vi "dB_autoselector.vi"(8 "error_in":errorcluster, 11 "Amplitude":dbl) -> (0 "error_out":errorcluster, 3 "Attenuator(dB)":T1)   [LabVIEW 2017]
uses:
  controls/attenuator_dB.ctl
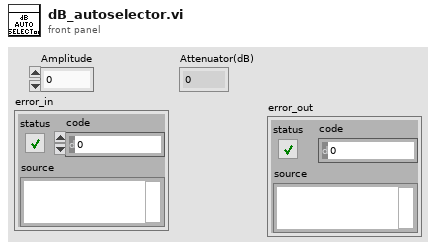
[diagram p1: front panel]
types:
  T1 = typedef "attenuator_dB.ctl" = enum16{"0", "20", "40", "60"}
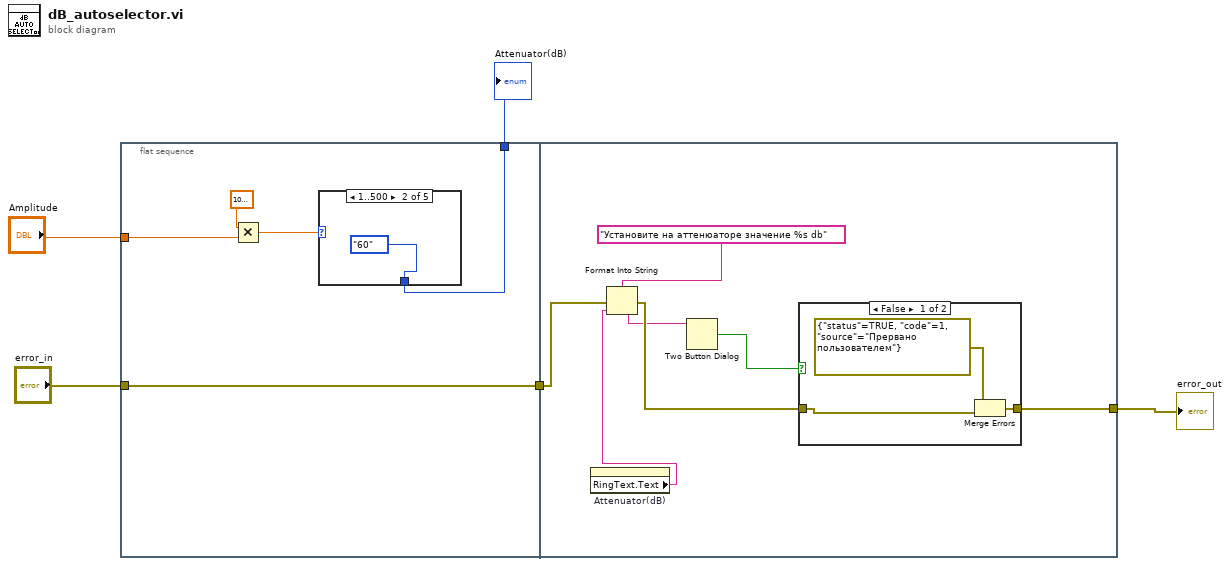
[diagram p0: block diagram]
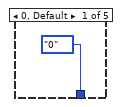
[diagram p2: hidden frame]
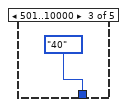
[diagram p3: hidden frame]
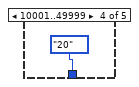
[diagram p4: hidden frame]
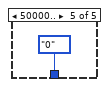
[diagram p5: hidden frame]
diagram:
  n1 = flat-sequence {
    tunnel: "error_in" -> [w8]
    tunnel: [w8] -> w4
    tunnel: "Amplitude" -> [w7]
    tunnel: [w6] -> w2
    tunnel: w4 -> [w18]
    tunnel: [w16] -> w1
    frame #0 {
      n2 = Multiply(x=1000000.0, y=w7) -> (x*y=w10:dbl)
      n3 = case shown="1..500" w10 {
        tunnel: [attenuator_dB."0" ("Attenuator(dB)") attenuator_dB."60" ("Attenuator(dB)") attenuator_dB."40" ("Attenuator(dB)") attenuator_dB."20" ("Attenuator(dB)") attenuator_dB."0" ("Attenuator(dB)")] -> w6
        frame 0, Default {
        }
        frame 1..500 {
        }
        frame 501..10000 {
        }
        frame 10001..49999 {
        }
        frame 50000.. {
        }
      }
    }
    frame #1 {
      n4 = property on="Attenuator(dB)" class="Enum (strict)"() -> ("RingText.Text"=w17:string)  [unwired: 2 in, 2 out]
      n5 = Format Into String(format string="Установите на аттенюаторе значение %s db", error in=w18, w17) -> (resulting string=w20:string, error out=w22:errorcluster)  [unwired: 1 in]
      n6 = Two Button Dialog(message=w20) -> (T button?=w21:bool)  [unwired: 2 in]
      n7 = case shown="False" w21 {
        tunnel: w22 -> [w23 w26]
        tunnel: [w25 w26] -> w16
        frame False {
          n8 = Merge Errors(errorcluster {"status"=TRUE, "code"=1, "source"="Прервано пользователем"} ("error constant"), w23) -> (w25:errorcluster)
        }
        frame True {
        }
      }
    }
  }
  "Attenuator(dB)" <- w2
  "error_out" <- w1
